vi "HV Load Test_Single Shot.vi"(5 "Published_Data_ID":string="HV39_", 10 "HV_Load_Steps_uA":dbl[](array[numeric])=[0.0, 5.0, 8.0, 10.0] format="%#_6p", 11 "Semiconductor Module Context":T1) -> (0 "error out":errorcluster)   [LabVIEW 2013]
uses:
  <vilib>/NI_TestStand_SemiconductorModule/NI_TestStand_Semiconductor_Module.lvlibp/PinMap/General/SemiconductorModuleContext.ctl
  <vilib>/NI_TestStand_SemiconductorModule/NI_TestStand_Semiconductor_Module.lvlibp/PinMap/DC Power/PinsToNIDCPowerSessions.vi
  <vilib>/NI_TestStand_SemiconductorModule/NI_TestStand_Semiconductor_Module.lvlibp/PinMap/General/Publish/PublishDataDouble2D.vi
  <vilib>/NI_TestStand_SemiconductorModule/NI_TestStand_Semiconductor_Module.lvlibp
panel:
  out "current measurements":dbl[][](array[numeric]) format="%#_6p"
  out "voltage measurements":dbl[][](array[numeric])
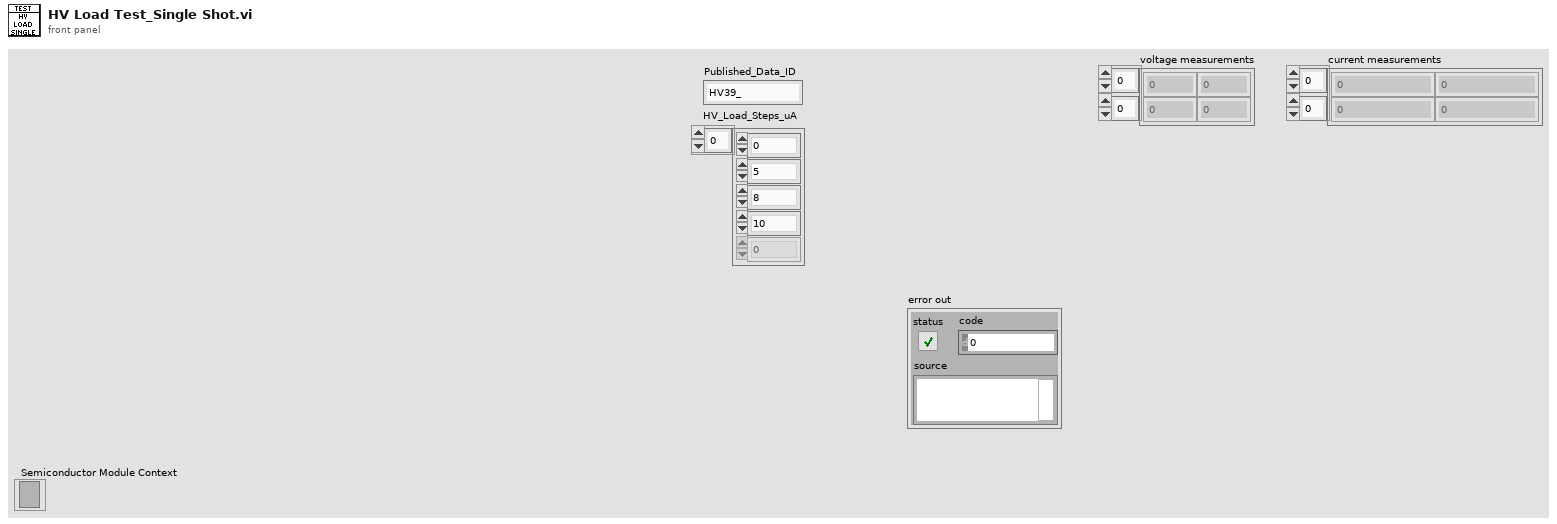
[diagram p1: front panel]
types:
  T1 = typedef "NI_TestStand_Semiconductor_Module.lvlibp/SemiconductorModuleContext.ctl" = refnum<k7>
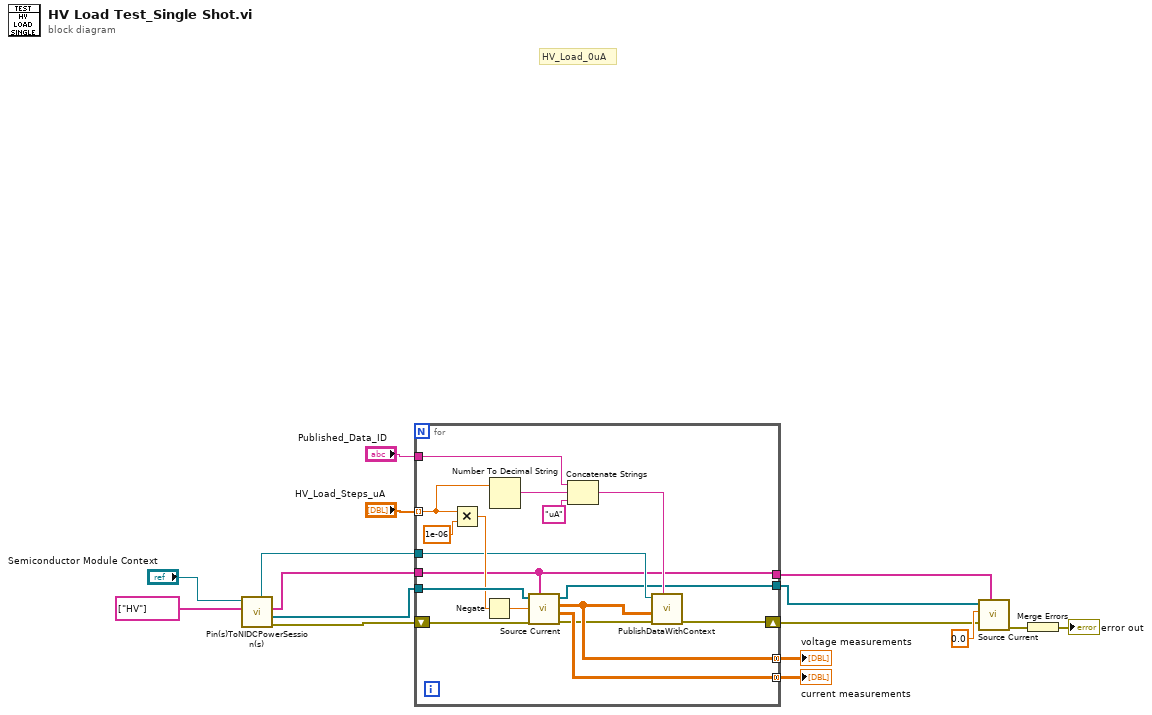
[diagram p0: block diagram]
diagram:
  # "HV_Load_0uA"
  n1 = call-poly <vilib>:"Pin(s)ToNIDCPowerSession(s).vi"("Pins"=string[] ["HV"], "Semiconductor Module Context"="Semiconductor Module Context") -> ("error out"=w13:errorcluster, "Instrument Sessions"=w14:refnum<k15>[], "Channel Lists"=w10:string[], "Pin Query Context"=w3:refnum<class "MultiplePinMultipleSessionQueryContext.lvclass">)  [unwired: 5 in, 1 out]
  n2 = for {
    tunnel: w10 -> [w17]
    tunnel: "HV_Load_Steps_uA" -> [w27] mode=indexing
    tunnel: w14 -> [w29]
    shift-right: [w21] -> w4
    shift-left: w13 -> [w30]
    tunnel: "Published_Data_ID" -> [w26]
    tunnel: [w23] -> w9 mode=concatenating
    tunnel: [w31] -> w7 mode=concatenating
    tunnel: w3 -> [w19]
    tunnel: [w18] -> w2
    tunnel: [w17] -> w1
    n3 = Multiply(x=w27, y=1e-06) -> (x*y=w28:dbl)
    n4 = Negate(x=w28) -> (-x=w32:dbl)
    n5 = Number To Decimal String(number=w27) -> (decimal integer string=w24:string)  [unwired: 1 in]
    n6 = call "Source Current.vi"("Channel Lists"=w17, "error in (no error)"=w30, "current level"=w32, "Instrument Sessions In"=w29) -> ("error out"=w22:errorcluster, "current measurements"=w31:dbl[][], "voltage measurements"=w23:dbl[][], "Instrument Sessions Out"=w18:refnum<k15>[])  [unwired: 4 in]
    n7 = Concatenate Strings(w26, w24, "uA" ("string")) -> (w20:string)
    n8 = call-poly <vilib>:"PublishDataWithContext.vi"("Published Data Id"=w20, "error in (no error)"=w22, "Data In"=w23, "Pin Query Context"=w19) -> ("error out"=w21:errorcluster)  [unwired: 6 in, 1 out]
  }
  "voltage measurements" <- w9
  "current measurements" <- w7
  n9 = call "Source Current.vi"("Channel Lists"=w1, "error in (no error)"=w4, "current level"=0.0, "Instrument Sessions In"=w2) -> ("error out"=w5:errorcluster)  [unwired: 4 in, 3 out]
  n10 = Merge Errors(w5) -> (→"error out":errorcluster)
